vi "GUARDADO_SIMULACION.vi"() -> ()   [LabVIEW 2019]
uses:
  <vilib>/drjdpowell/SQLite Library/SQL Connection/Open (path).vi
  <vilib>/drjdpowell/SQLite Library/SQL Connection/Open (string).vi
  <vilib>/AdvancedString/Path To Command Line String.vi
  <vilib>/drjdpowell/SQLite Library/SQL Connection/Execute SQL.vi
  <vilib>/drjdpowell/SQLite Library/SQL Connection/Connection.lvclass
  <vilib>/drjdpowell/SQLite Library/SQLite.lvlib
panel:
  in  "stop":bool
  out "appended array":string[][](array[string])
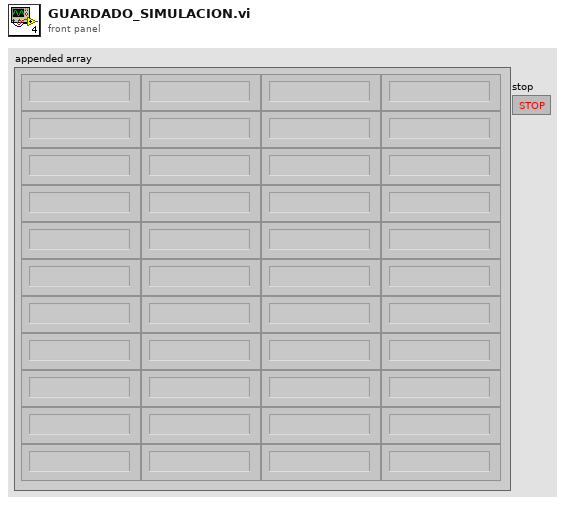
[diagram p1: front panel]
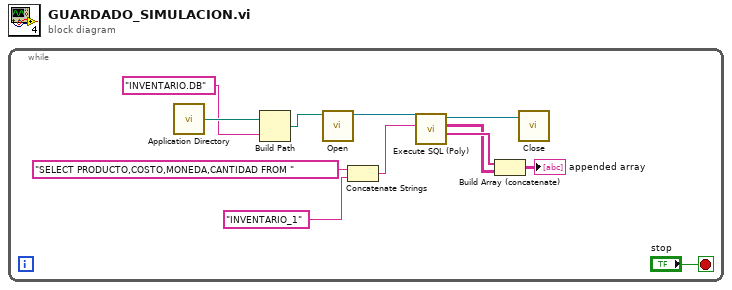
[diagram p0: block diagram]
diagram:
  n1 = while {
    stop <- "stop" stop-if-true
    n2 = call <vilib>:"Application Directory.vi"() -> ("Application Directory"=w12:path)
    n3 = Build Path(base path=w12, name or relative path="INVENTARIO.DB") -> (appended path=w11:path)
    n4 = call-poly <vilib>:"Open.vi"("db file"=w11) -> ("SQLite Connection"=w10:refnum<class "Connection.lvclass">)  [unwired: 9 in, 1 out]
    n5 = Concatenate Strings("SELECT PRODUCTO,COSTO,MONEDA,CANTIDAD FROM " ("string"), "INVENTARIO_1" ("string")) -> (w7:string)
    n6 = call-poly <vilib>:"Execute SQL (Poly).vi"("SQL"=w7, "SQLite Connection in"=w10) -> ("Column Names"=w6:string[], "Result Set"=w5:string[][], "SQLite Connection"=w9:refnum<class "Connection.lvclass">)  [unwired: 6 in, 1 out]
    n7 = Build Array (concatenate)(w6, w5) -> (→"appended array":string[][])
    n8 = call-dynamic "Close.vi"("SQLite Connection in"=w9) -> ()  [unwired: 10 in, 1 out]
  }
